vi "Add Channel.vi"(5 "Action":T2, 7 "SysDef Name":string, 8 "error in (no error)":errorcluster, 10 "Register Index":i32, 11 "Node Ptr in":T1 format="%.0x") -> (0 "error out":errorcluster, 3 "Node Ptr out":T1=18446744073709551615 format="%.0x")   [LabVIEW 2019, in "Scripting API.lvlib"]
uses:
  Scripting API.lvlib
  Addon/Addon System Explorer/Types/Channel Type.ctl
  <vilib>/NI VeriStand/Custom Device API/Custom Device Item Ref.ctl
  Addon/Addon Shared/Types/FG Action.ctl
  Addon/Addon Shared/SubVIs/Constants.vi
  <vilib>/NI/NI VeriStand Advanced SysDef API/SysDef API/SysDef.Property.Get.vi
  <vilib>/NI/NI VeriStand Advanced SysDef API/_SubVIs/SysDef.Property.Get.Variant.vi
  <vilib>/NI/NI VeriStand Advanced SysDef API/SysDef API/SysDef.Property.Set.vi
  <vilib>/NI/NI VeriStand Advanced SysDef API/_SubVIs/SysDef.Property.Set.Variant.vi
  Addon/Addon Shared/FPGA Addon Shared.lvlib
  Addon/Addon System Explorer/FPGA Addon System Explorer.lvlib
  <vilib>/NI VeriStand/Custom Device API/Custom Device API.lvlib
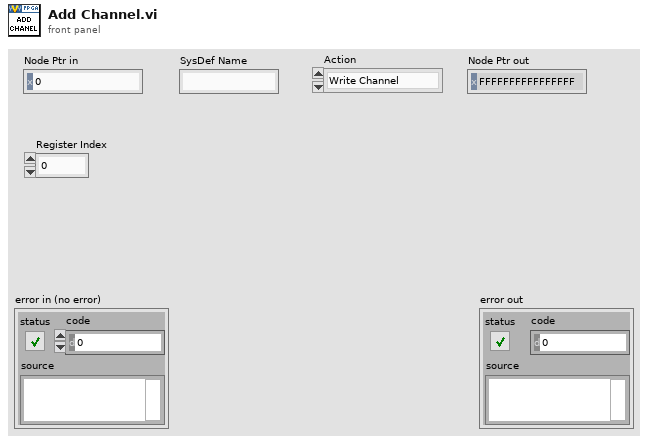
[diagram p1: front panel]
types:
  T1 = typedef "Custom Device API.lvlib/Custom Device Item Ref.ctl" = u64
  T2 = typedef "FPGA Addon System Explorer.lvlib/Channel Type.ctl" = enum16{"Write Channel", "Read Channel", "Write Waveform", "Read Waveform"}
  T3 = typedef "FPGA Addon Shared.lvlib/FG Action.ctl" = enum8{"GET", "SET"}
  T4 = typedef "FPGA Addon Shared.lvlib/Register Information.ctl" = cluster{"Name":string, "Data Type":T5, "Default Value":variant, "Attributes":variant}
  T5 = typedef "FPGA Addon Shared.lvlib/FPGA Addon Data Type.ctl" = enum8{"<Null>", "I8", "I16", "I32", "I64", "U8", "U16", "U32", "U64", "SGL", "Boolean", "Analog PWM In Settings", "Analog PWM In", "Digital PWM In Settings", "Digital PWM In", "Digital PWM Out", "Sine Out", "FXP", "FXP+/-24.5", "FXP+/-16.5", "FXP+/-32.8", "FXP+/-64.32", "FXP+/-16.7", "FXP+/-20.5", "FXP+/-27.5", "FXP+/-32.16", "FXP+16.3", "FXP+18.3", "Digital Static In", "Digital Static Out", "Digital Static In Settings", "Digital WSS Out", "Quad Encoder Settings", "Quad Encoder In", "Group"}
  T6 = typedef "FPGA Addon Shared.lvlib/DMA Information.ctl" = cluster{"Name":string, "Data Type":T5}
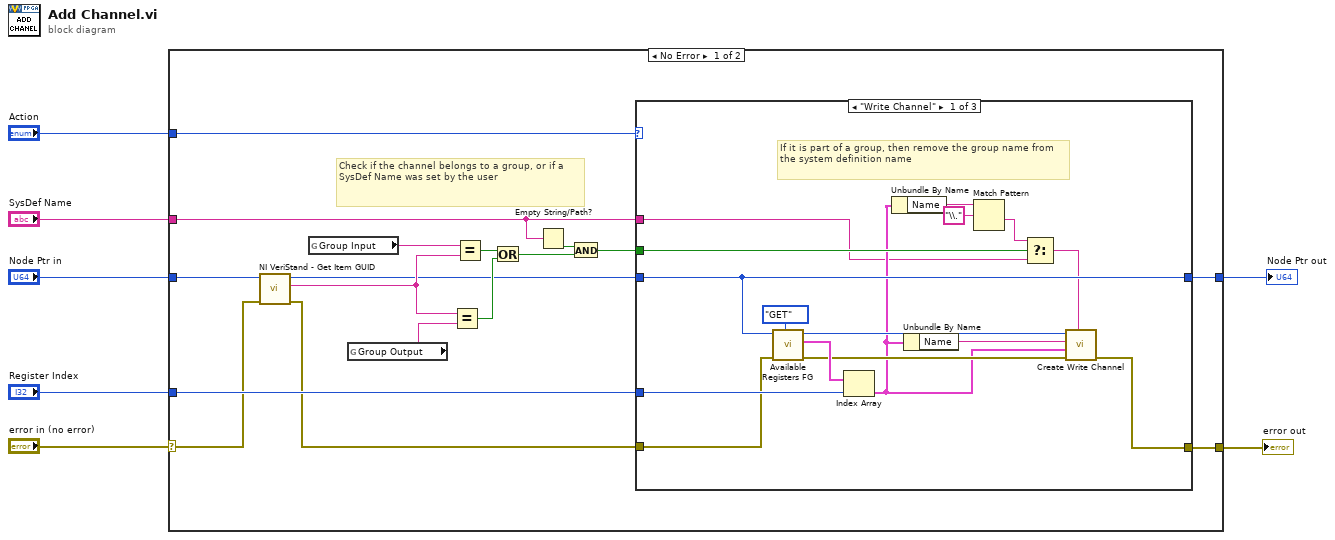
[diagram p0: block diagram]
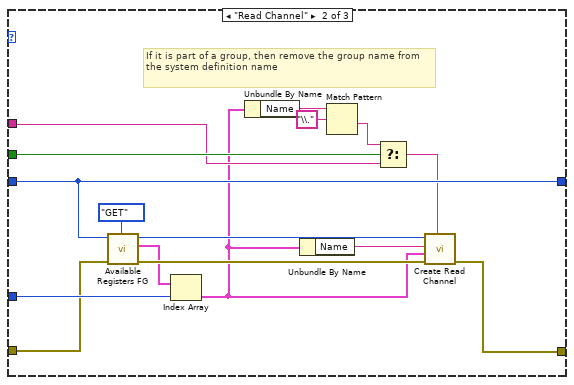
[diagram p2: hidden frame]
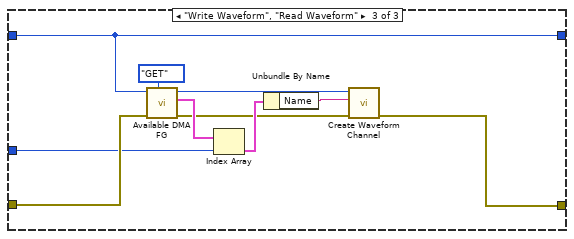
[diagram p3: hidden frame]
diagram:
  n1 = case shown="No Error" "error in (no error)" {
    selector: "error in (no error)" -> [w19 w67]
    tunnel: [w24 w67] -> w7
    tunnel: "Action" -> [w23 _]
    tunnel: "Register Index" -> [w22 _]
    tunnel: "Node Ptr in" -> [w20 w68]
    tunnel: "SysDef Name" -> [w11 _]
    tunnel: [w21 w68] -> w2
    frame No Error {
      # "Check if the channel belongs to a group, or if a SysDef Name was set by the user"
      n2 = call <vilib>:"NI VeriStand - Get Item GUID.vi"("error in (no error)"=w19, "Item Ref in"=w20) -> ("error out"=w18:errorcluster, "GUID"=w16:string, "Item Ref out"=w12:T1)  [unwired: 7 in]
      n3 = global read "Constants.vi" "Group Input"() -> (w15:string)
      n4 = global read "Constants.vi" "Group Output"() -> (w17:string)
      n5 = Equal?(x=w16, y=w17) -> (x = y?=w14:bool)
      n6 = Equal?(x=w15, y=w16) -> (x = y?=w13:bool)
      n7 = Or(x=w13, y=w14) -> (x .or. y?=w9:bool)
      n8 = Empty String/Path?(string/path=w11) -> (empty?=w10:bool)
      n9 = And(x=w10, y=w9) -> (x .and. y?=w8:bool)
      n10 = case shown="\"Write Channel\"" w23 {
        tunnel: [w36 w50 w66] -> w24
        tunnel: w12 -> [w32 w49 w58]
        tunnel: w22 -> [w37 w53 w63]
        tunnel: w18 -> [w34 w51 w65]
        tunnel: w11 -> [w26 w43 _]
        tunnel: [w32 w49 w58] -> w21
        tunnel: w8 -> [w28 w46 _]
        frame "Write Channel" {
          # "If it is part of a group, then remove the group name from the system definition name"
          n11 = call "Available Registers FG.vi"("Action"=FG_Action."GET", "error in (no error)"=w34, "Item Ref"=w32) -> ("error out"=w38:errorcluster, "Available Registers"=w39:T4[], "Item Ref out"=w35:T1)  [unwired: 6 in]
          n12 = Index Array(array=w39, index=w37) -> (element=w27:T4)
          n13 = Unbundle By Name(w27) -> ("Name"=w31:string)
          n14 = Unbundle By Name(w27) -> ("Name"=w33:string)
          n15 = Match Pattern(string=w31, regular expression="\\.") -> (after substring=w29:string)  [unwired: 1 in, 3 out]
          n16 = Select(t=w29, s=w28, f=w26) -> (s? t:f=w25:string)
          n17 = call "Create Write Channel.vi"("Name"=w25, "error in (no error)"=w38, "Cluster"=w27, "Bitfile Name"=w33, "Item Ref in"=w35) -> ("error out"=w36:errorcluster)  [unwired: 6 in]
        }
        frame "Read Channel" {
          # "If it is part of a group, then remove the group name from the system definition name"
          n18 = call "Available Registers FG.vi"("Action"=FG_Action."GET", "error in (no error)"=w51, "Item Ref"=w49) -> ("error out"=w55:errorcluster, "Available Registers"=w54:T4[], "Item Ref out"=w52:T1)  [unwired: 6 in]
          n19 = Index Array(array=w54, index=w53) -> (element=w42:T4)
          n20 = Unbundle By Name(w42) -> ("Name"=w48:string)
          n21 = Unbundle By Name(w42) -> ("Name"=w41:string)
          n22 = Match Pattern(string=w48, regular expression="\\.") -> (after substring=w45:string)  [unwired: 1 in, 3 out]
          n23 = Select(t=w45, s=w46, f=w43) -> (s? t:f=w44:string)
          n24 = call "Create Read Channel.vi"("Name"=w44, "error in (no error)"=w55, "Channel"=w42, "Bitfile Name"=w41, "Item Ref in"=w52) -> ("error out"=w50:errorcluster)  [unwired: 6 in]
        }
        frame "Write Waveform", "Read Waveform" {
          n25 = call "Available DMA FG.vi"("Action"=FG_Action."GET", "error in (no error)"=w65, "Item Ref"=w58) -> ("error out"=w59:errorcluster, "Available DMA"=w64:T6[], "Item Ref out"=w62:T1)  [unwired: 6 in]
          n26 = Index Array(array=w64, index=w63) -> (element=w61:T6)
          n27 = Unbundle By Name(w61) -> ("Name"=w60:string)
          n28 = call "Create Waveform Channel.vi"("error in (no error)"=w59, "Bitfile Name"=w60, "Item Ref in"=w62) -> ("error out"=w66:errorcluster)  [unwired: 8 in]
        }
      }
    }
    frame Error {
    }
  }
  "error out" <- w7
  "Node Ptr out" <- w2
